vi "_Axis_SetV.vi"(8 "Error In":errorcluster, 10 "最大速度":i32, 11 "轴序号":u16) -> (0 "Error Out":errorcluster)   [LabVIEW 2020, in "MT_API.lvlib"]
doc: "MT_API INT32 __stdcall MT_Set_Axis_Position_V_Max(WORD AObj,INT32 Value);"
uses:
  MT_API.lvlib
  MT_API_64.dll
panel:
  out "函数返回值":i32
  # "设置位置模式下轴最大移动速度"
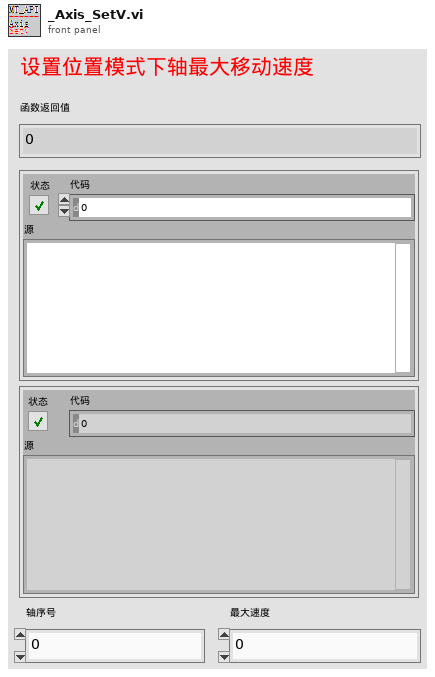
[diagram p1: front panel]
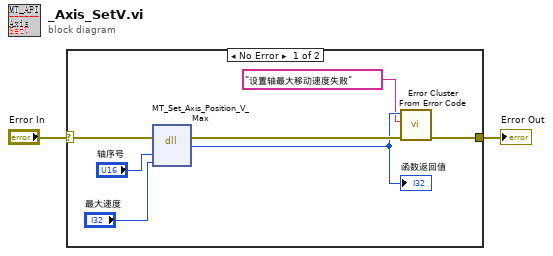
[diagram p0: block diagram]
diagram:
  n1 = case shown="No Error" "Error In" {
    selector: "Error In" -> [w8 w10]
    tunnel: [w7 w10] -> w1
    frame No Error {
      n2 = dll-call lib="D:/Project NJU/lib/MT/MT_API_64.*" fn="MT_Set_Axis_Position_V_Max"(error in=w8, "AObj"="轴序号", "Value"="最大速度") -> (error out=w9:errorcluster, "return type"=w6:i32)  [unwired: 4 in, 1 out]
      "函数返回值" <- w6
      n3 = call <vilib>:"Error Cluster From Error Code.vi"("error in (no error)"=w9, "error message (\"\")"="设置轴最大移动速度失败", "error code (0)"=w6) -> ("error out"=w7:errorcluster)  [unwired: 6 in]
    }
    frame Error {
    }
  }
  "Error Out" <- w1
